vi "Read Comp Driver Config.vi"(8 "error in (no error)":errorcluster, 11 "Comp Driver in":refnum<class "Comp Driver.lvclass">) -> (0 "error out":errorcluster, 2 "Comp Driver Config":T1, 3 "Comp Driver out":refnum<class "Comp Driver.lvclass">)   [LabVIEW 2014, in "Comp Driver.lvlib" / "Comp Driver.lvclass"]
uses:
  Comp Driver.lvclass
  Comp Driver Config.ctl
  <vilib>/Rock Robotics/WPI/Joystick/WPI_JoystickDeviceEnum.ctl
  Comp Driver.lvclass/Comp Driver.ctl
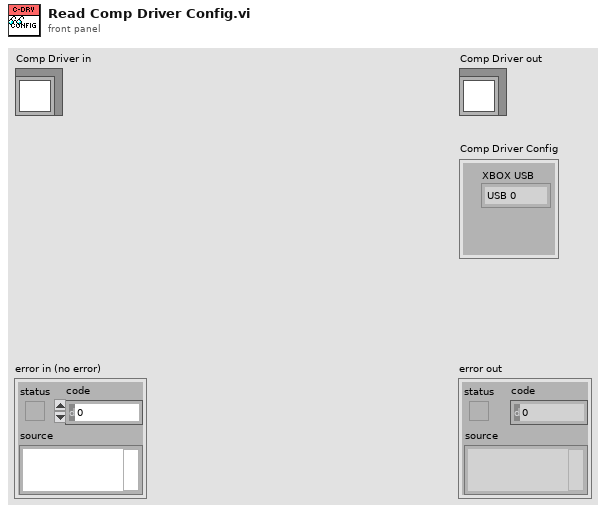
[diagram p1: front panel]
types:
  T1 = typedef "Comp Driver.lvlib/Comp Driver.lvclass/Comp Driver Config.ctl" = cluster{"XBOX USB":T2}
  T2 = typedef "WPI_JoystickDeviceEnum.ctl" = enum16{"USB 0", "USB 1", "USB 2", "USB 3", "USB 4", "USB 5"}
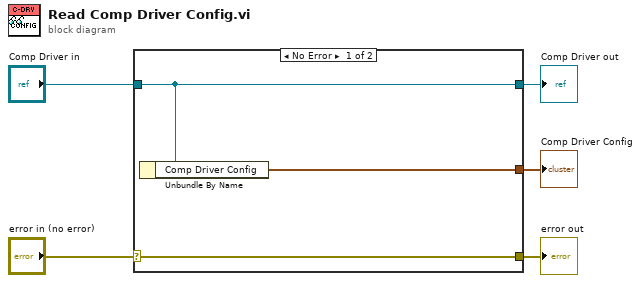
[diagram p0: block diagram]
diagram:
  n1 = case shown="No Error" "error in (no error)" {
    selector: "error in (no error)" -> [w8 w9]
    tunnel: [w8 w9] -> w4
    tunnel: [w7 w10] -> w2
    tunnel: "Comp Driver in" -> [w7 w10]
    tunnel: [w6 _] -> w1
    frame No Error {
      n2 = Unbundle By Name(w7) -> ("Comp Driver Config"=w6:T1)
    }
    frame Error {
    }
  }
  "error out" <- w4
  "Comp Driver out" <- w2
  "Comp Driver Config" <- w1
